vi "Check Count.vi"(5 "source vi name":string, 6 "count power of 2":u8, 7 "buffer count":u64 format="%d elements", 8 "error in (no error)":errorcluster, 9 "offset (0)":u64 format="%d bytes", 10 "count (-1: rest)":i64=-1 format="%d elements", 11 "Pointer in":refnum<class "Pointer.lvclass">) -> (0 "error out":errorcluster, 1 "offset":u64 format="%d bytes", 2 "count":u64 format="%d elements", 3 "Pointer out":refnum<class "Pointer.lvclass">)   [LabVIEW 2027, in "Memory Manager.lvlib" / "Pointer.lvclass"]
uses:
  Pointer.lvclass
  Out of Bounds.vi
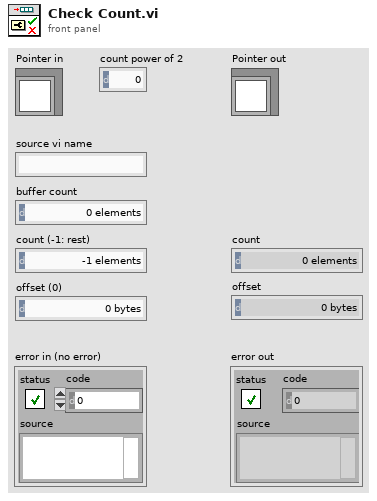
[diagram p1: front panel]
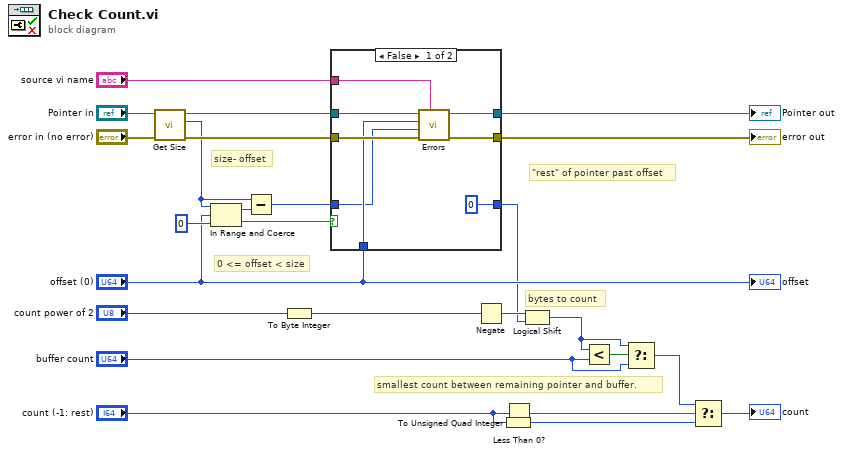
[diagram p0: block diagram]
diagram:
  # "smallest count between remaining pointer and buffer."
  # "\"rest\" of pointer past offset"
  # "bytes to count"
  # "size- offset"
  # "0 <= offset < size"
  n1 = call "Get Size.vi"("Pointer in"="Pointer in") -> ("size"=w13:u64, "Pointer out"=w19:refnum<class "Pointer.lvclass">)  [unwired: 9 in]
  n2 = In Range and Coerce(upper limit=w13, x="offset (0)", lower limit=u64 0) -> (coerced(x)=w12:u64, In Range?=w20:bool)
  n3 = Subtract(x=w13, y=w12) -> (x-y=w11:u64)
  n4 = To Byte Integer(number="count power of 2") -> (8bit integer=w1:i8)
  n5 = case shown="False" w20 {
    tunnel: w19 -> [w32 w35]
    tunnel: "error in (no error)" -> [w31 w34]
    tunnel: [w30 w35] -> w17
    tunnel: [w29 w34] -> w16
    tunnel: "source vi name" -> [w28 _]
    tunnel: "offset (0)" -> [w27 _]
    tunnel: w11 -> [w26 w33]
    tunnel: [u64 0 ("t") w33] -> w9
    frame False {
      n6 = call-poly "Errors.vi"("error source vi name"=w28, "error in (no error)"=w31, "size"=w26, "offset"=w27, "Pointer in"=w32) -> ("error out"=w29:errorcluster, "Pointer out"=w30:refnum<class "Pointer.lvclass">)  [unwired: 5 in]
    }
    frame True {
    }
  }
  "error out" <- w16
  "Pointer out" <- w17
  n7 = Negate(x=w1) -> (-x=w14:i8)
  n8 = To Unsigned Quad Integer(1:"count (-1: rest)") -> (0:w23:u64)
  n9 = Less Than 0?(x="count (-1: rest)") -> (x < 0?=w22:bool)
  n10 = Logical Shift(y=w14, x=w9) -> (x << y=w4:u64)
  n11 = Less?(x=w4, y="buffer count") -> (x < y?=w6:bool)
  n12 = Select(t=w4, s=w6, f="buffer count") -> (s? t:f=w3:u64)
  n13 = Select(t=w3, s=w22, f=w23) -> (s? t:f=→"count":u64)
  "offset" <- "offset (0)"
